vi "Get All RFSG Sessions and Tester Info with Tester Type.vi"(0 "TSM Context In":T1, 5 "Tester Type":string="RFPM", 11 "error in":errorcluster) -> (4 "TSM Context Out":T1, 6 "RFSG Sessions":refnum<k15>[](array[refnum]), 8 "Resource Descriptors":string[](array[string]), 10 "Instrument Models":string[](array[string]), 15 "error out":errorcluster)   [LabVIEW 2023, in "RFCalAndFixtureCharact.Common.lvlib"]
uses:
  RFCalAndFixtureCharact.Common.lvlib
  <vilib>/NI_TestStand_SemiconductorModule/NI_TestStand_Semiconductor_Module.lvlibp
  <vilib>/ErrorRing/Error Ring.xnode
  <vilib>/Utility/error.llb/Error Cluster From Error Code.vi
  <vilib>/NI_TestStand_SemiconductorModule/NI_TestStand_Semiconductor_Module.lvlibp/PinMap/General/SemiconductorModuleContext.ctl
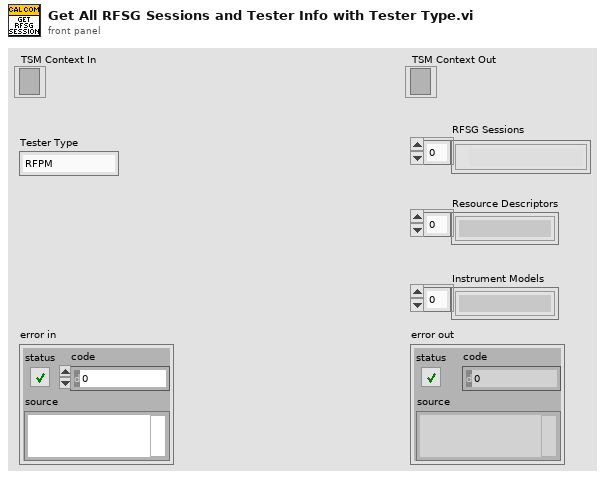
[diagram p1: front panel]
types:
  T1 = typedef "NI_TestStand_Semiconductor_Module.lvlibp/SemiconductorModuleContext.ctl" = refnum<k7>
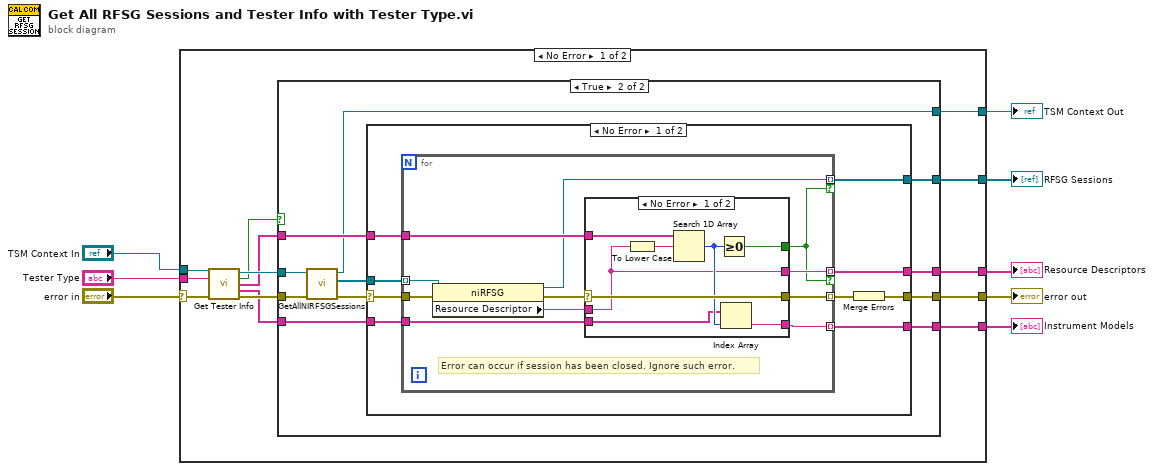
[diagram p0: block diagram]
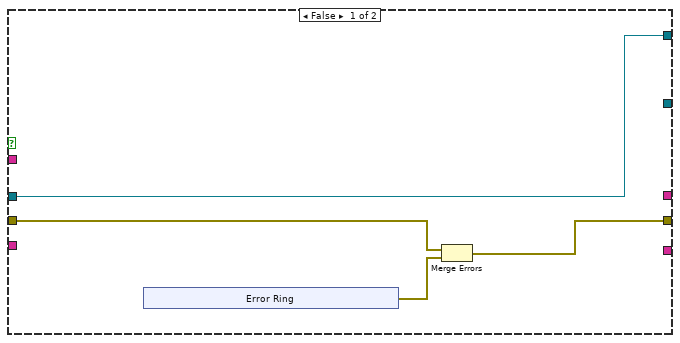
[diagram p2: hidden frame]
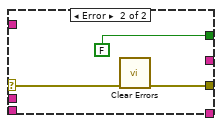
[diagram p3: hidden frame]
diagram:
  n1 = case shown="No Error" "error in" {
    selector: "error in" -> [w14 w75]
    tunnel: "TSM Context In" -> [w21 w74]
    tunnel: [w20 w75] -> w7
    tunnel: [w19 _] -> w6
    tunnel: "Tester Type" -> [w18 _]
    tunnel: [w15 w74] -> w4
    tunnel: [w12 _] -> w2
    tunnel: [w11 _] -> w1
    frame No Error {
      n2 = call "Get Tester Info.vi"("TSM Context In"=w21, "Tester Type"=w18, "error in"=w14) -> ("TSM Context Out"=w16:T1, "Resource Descriptors Exist?"=w10:bool, "Resource Descriptors"=w9:string[], "Instrument Models"=w13:string[], "error out"=w17:errorcluster)  [unwired: 8 in]
      n3 = case shown="True" w10 {
        tunnel: w9 -> [_ w41]
        tunnel: w17 -> [w25 w38]
        tunnel: [w23 w40] -> w20
        tunnel: [_ w39] -> w19
        tunnel: w16 -> [w22 w35]
        tunnel: [w22 w34] -> w15
        tunnel: w13 -> [_ w33]
        tunnel: [_ w32] -> w12
        tunnel: [_ w31] -> w11
        frame False {
          n4 = xnode "Error Ring"() -> ("error out"=w24:errorcluster)
          n5 = Merge Errors(w25, w24) -> (w23:errorcluster)
        }
        frame True {
          n6 = call <vilib>:"GetAllNIRFSGSessions.vi"("error in (no error)"=w38, "Semiconductor Module Context"=w35) -> ("error out"=w37:errorcluster, "Instrument Sessions"=w36:refnum<k15>[], "Semiconductor Module Context Out"=w34:T1)  [unwired: 7 in]
          n7 = case shown="No Error" w37 {
            selector: w37 -> [w48 w73]
            tunnel: w36 -> [w50 _]
            tunnel: w41 -> [w49 _]
            tunnel: [w46 w73] -> w40
            tunnel: [w45 _] -> w39
            tunnel: w33 -> [w44 _]
            tunnel: [w43 _] -> w32
            tunnel: [w42 _] -> w31
            frame No Error {
              n8 = for {
                tunnel: w48 -> [w56]
                tunnel: w50 -> [w57] mode=indexing
                tunnel: w49 -> [w59]
                tunnel: [w55] -> w45 mode=indexing if=w51
                tunnel: [w58] -> w47 mode=indexing
                tunnel: w44 -> [w54]
                tunnel: [w53] -> w43 mode=indexing
                tunnel: [w52] -> w42 mode=indexing if=w51
                # "Error can occur if session has been closed. Ignore such error."
                n9 = property class="niRFSG"(reference=w57, error in=w56) -> (reference out=w55:refnum<k15>, error out=w61:errorcluster, "Resource Descriptor"=w60:string)
                n10 = case shown="No Error" w61 {
                  selector: w61 -> [w67 w71]
                  tunnel: w60 -> [w62 _]
                  tunnel: w59 -> [w69 _]
                  tunnel: [w68 FALSE] -> w51
                  tunnel: [w67 w70] -> w58
                  tunnel: w54 -> [w64 _]
                  tunnel: [w63 _] -> w53
                  tunnel: [w62 _] -> w52
                  frame No Error {
                    n11 = To Lower Case(string=w62) -> (all lower case string=w66:string)
                    n12 = Search 1D Array(1D array=w69, element=w66) -> (index of element=w65:i32)  [unwired: 1 in]
                    n13 = Greater Or Equal To 0?(x=w65) -> (x >= 0?=w68:bool)
                    n14 = Index Array(array=w64, index=w65) -> (element=w63:string)
                  }
                  frame Error {
                    n15 = call <vilib>:"Clear Errors.vi"("error in (no error)"=w71) -> ("error out"=w70:errorcluster)  [unwired: 5 in, 1 out]
                  }
                }
              }
              n16 = Merge Errors(w47) -> (w46:errorcluster)
            }
            frame Error {
            }
          }
        }
      }
    }
    frame Error {
    }
  }
  "TSM Context Out" <- w4
  "error out" <- w7
  "RFSG Sessions" <- w6
  "Instrument Models" <- w2
  "Resource Descriptors" <- w1
